vi "1_Counter_Time_Trace.vi"() -> ()   [LabVIEW 2015]
uses:
  C:/Users/MX-Microscope/Documents/LabVIEW Data/lvoop_campus_2018/Detector_Class/Swabian/time_tagger_vis/TTCSharp32.dll
  TTCSharp32.dll
panel:
  out "XY Graph 2":cluster{"Y":dbl[], "Y":dbl[]}[](graph)
  out "XY Graph":cluster{"Y":dbl[], "Y":dbl[]}[](graph)
  # "The built in test signal (~ 800 to 900 kHz) is applied first to channel 0 and 1 s later to channel 1."
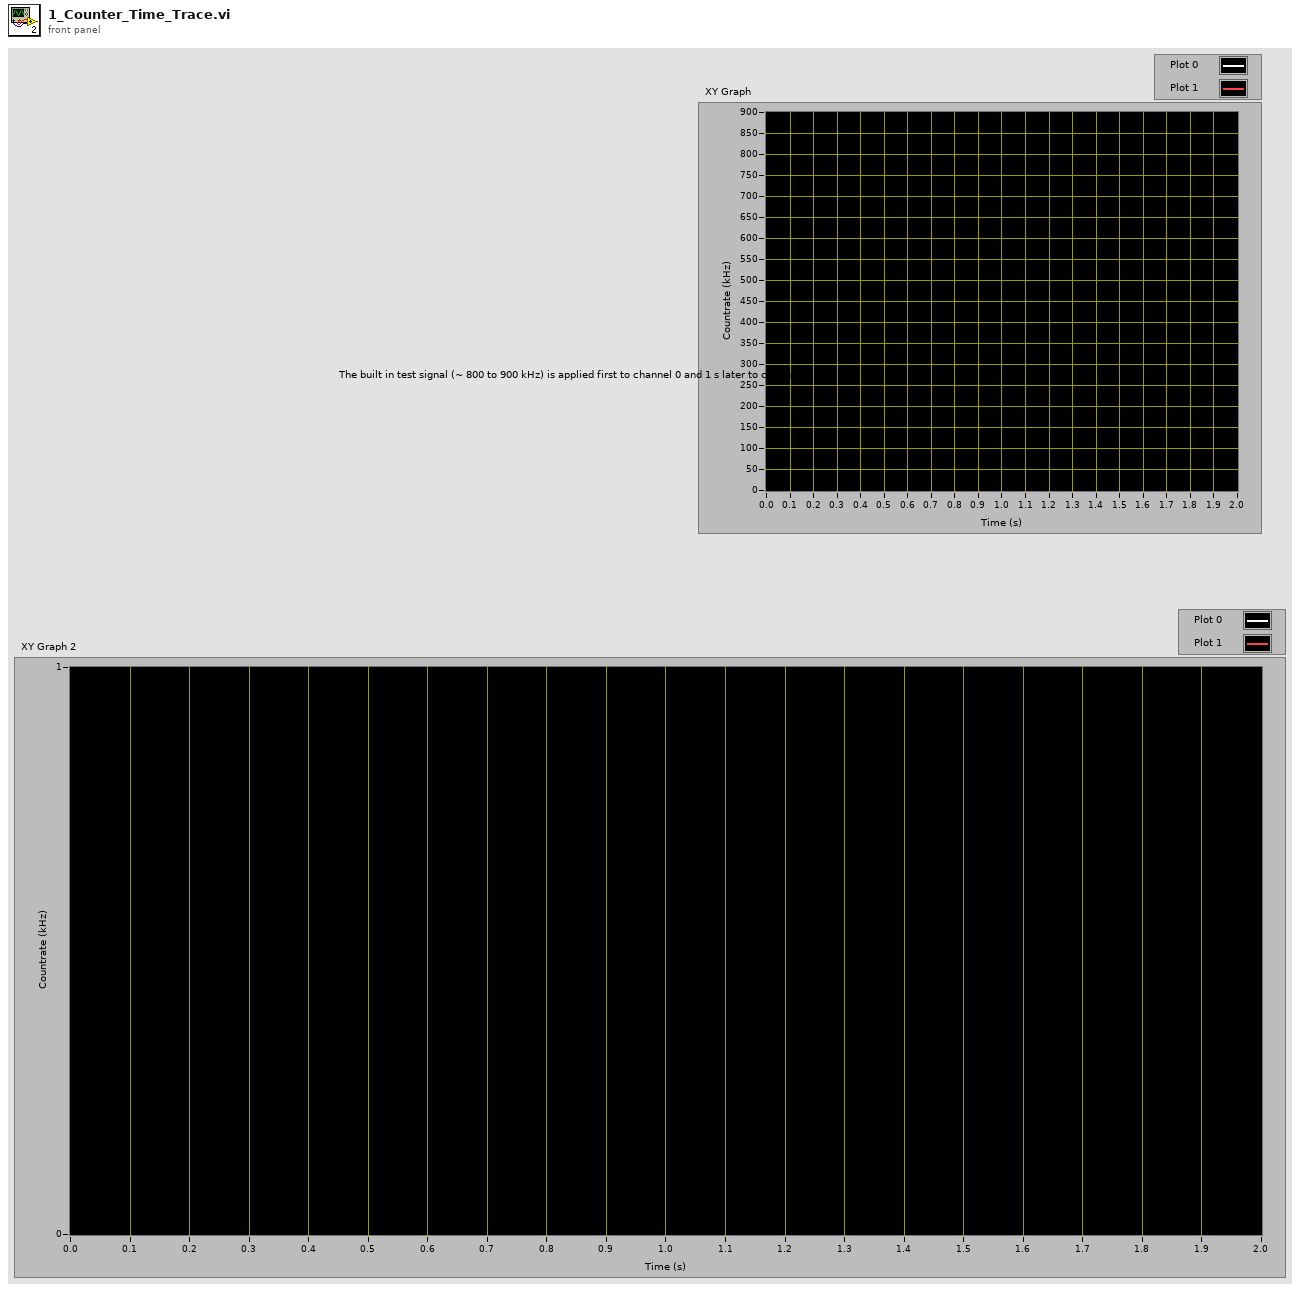
[diagram p1: front panel]
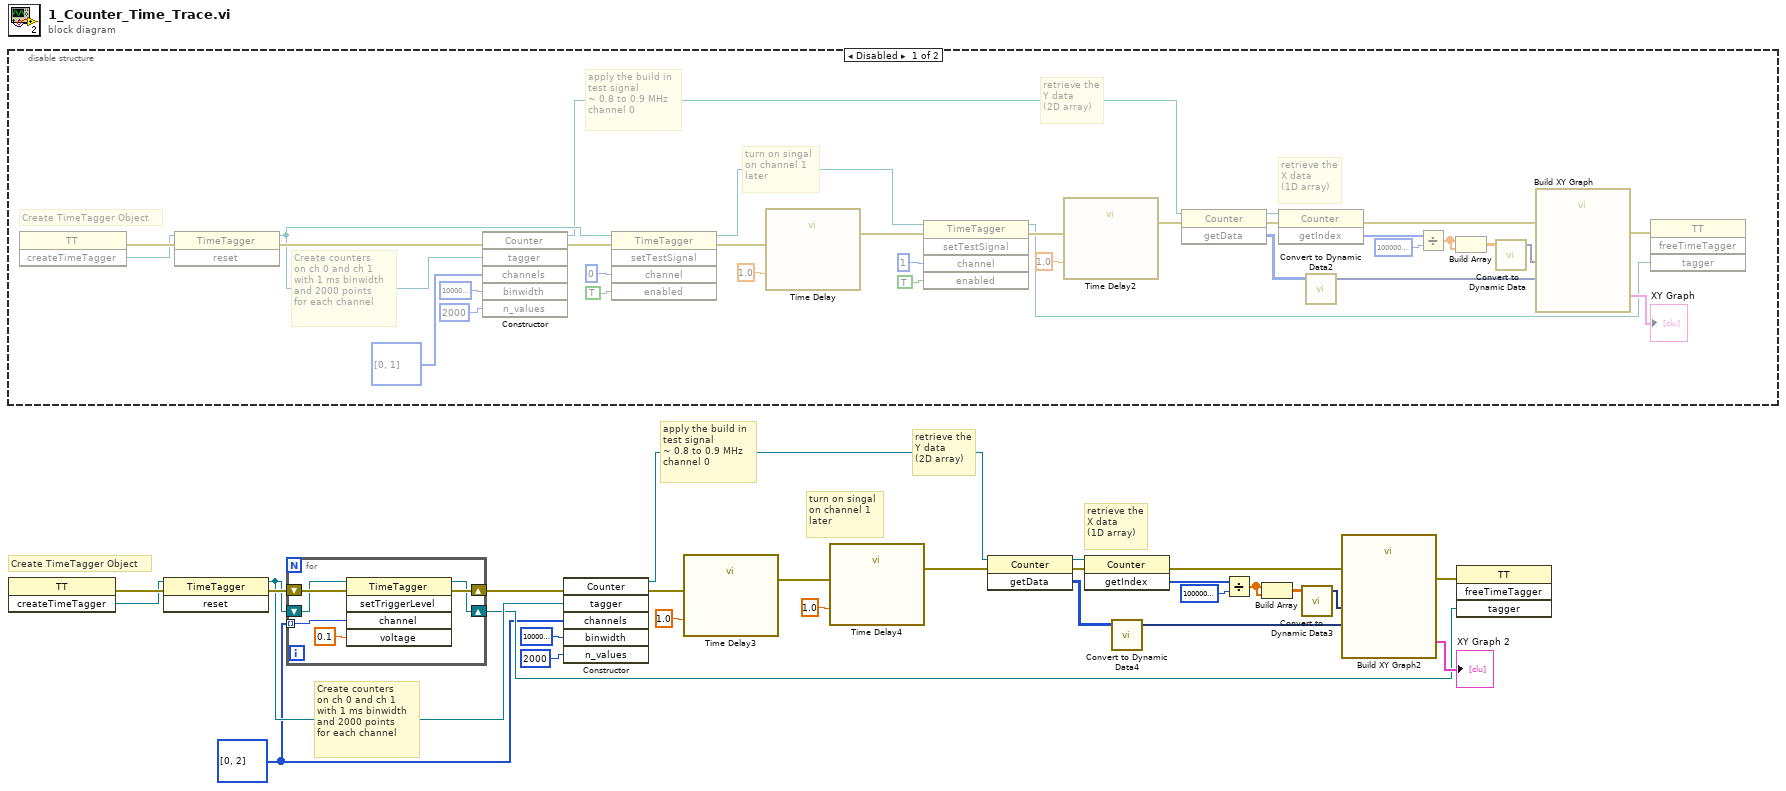
[diagram p0: block diagram]
diagram:
  w1 = u32[] [0, 2] ("channels")
  # "retrieve the\nX data\n(1D array)"
  # "retrieve the\nY data\n(2D array)"
  # "turn on singal\non channel 1\nlater"
  # "apply the build in\ntest signal\n~ 0.8 to 0.9 MHz\nchannel 0"
  # "Create counters\non ch 0 and ch 1\nwith 1 ms binwidth\nand 2000 points\nfor each channel"
  # "Create TimeTagger Object"
  n1 = disable-structure shown="Disabled" {
    frame Disabled {
      # "retrieve the\nX data\n(1D array)"
      # "retrieve the\nY data\n(2D array)"
      # "turn on singal\non channel 1\nlater"
      # "apply the build in\ntest signal\n~ 0.8 to 0.9 MHz\nchannel 0"
      # "Create counters\non ch 0 and ch 1\nwith 1 ms binwidth\nand 2000 points\nfor each channel"
      # "Create TimeTagger Object"
      n2 = invoke class="TT" method="createTimeTagger"() -> (error out=w56:errorcluster, "createTimeTagger"=w55:refnum<k24>)  [unwired: 3 in, 1 out]
      n3 = invoke class="TimeTagger" method="reset"(reference=w55, error in=w56) -> (reference out=w47:refnum<k24>, error out=w54:errorcluster)  [unwired: 1 in, 1 out]
      n4 = constructor class="Counter"(error in=w54, "tagger"=w47, "channels"=u32[] [0, 1], "binwidth"=i64 1000000000, "n_values"=2000) -> (reference out=w45:refnum<k24>, error out=w46:errorcluster)  [unwired: 2 in, 5 out]
      n5 = invoke class="TimeTagger" method="setTestSignal"(reference=w47, error in=w46, "channel"=u32 0, "enabled"=TRUE) -> (reference out=w48:refnum<k24>, error out=w50:errorcluster)  [unwired: 1 in, 3 out]
      n6 = call "Time Delay"("error in (no error)"=w50, "Delay Time (s)"=1.0) -> ("error out"=w49:errorcluster)  [unwired: 9 in]
      n7 = invoke class="TimeTagger" method="setTestSignal"(reference=w48, error in=w49, "channel"=u32 1, "enabled"=TRUE) -> (reference out=w28:refnum<k24>, error out=w43:errorcluster)  [unwired: 1 in, 3 out]
      n8 = call "Time Delay2"("error in (no error)"=w43, "Delay Time (s)"=1.0) -> ("error out"=w40:errorcluster)  [unwired: 9 in]
      n9 = invoke class="Counter" method="getData"(reference=w45, error in=w40) -> (reference out=w42:refnum<k24>, error out=w41:errorcluster, "getData"=w34:i32[][])  [unwired: 1 in]
      n10 = invoke class="Counter" method="getIndex"(reference=w42, error in=w41) -> (error out=w37:errorcluster, "getIndex"=w32:i64[])  [unwired: 1 in, 1 out]
      n11 = call "Convert to Dynamic Data2"("2D Array"=w34) -> ("Dynamic Data Type"=w33:dynamicdata)  [unwired: 3 in]
      n12 = Divide(x=w32, y=i64 1000000000000) -> (x/y=w31:dbl[])
      n13 = Build Array(w31, w31) -> (w36:dbl[][])
      n14 = call "Convert to Dynamic Data"("2D Array"=w36) -> ("Dynamic Data Type"=w35:dynamicdata)  [unwired: 3 in]
      n15 = call "Build XY Graph"("error in (no error)"=w37, "Y Input"=w33, "X Input"=w35) -> ("error out"=w29:errorcluster, "XY Graph"=→"XY Graph":cluster{"X":dbl[], "Y":dbl[]}[])  [unwired: 7 in]
      n16 = invoke class="TT" method="freeTimeTagger"(error in=w29, "tagger"=w28) -> ()  [unwired: 2 in, 4 out]
    }
    frame Enabled {
    }
  }
  n17 = invoke class="TT" method="createTimeTagger"() -> (error out=w27:errorcluster, "createTimeTagger"=w26:refnum<k24>)  [unwired: 3 in, 1 out]
  n18 = invoke class="TimeTagger" method="reset"(reference=w26, error in=w27) -> (reference out=w3:refnum<k24>, error out=w5:errorcluster)  [unwired: 1 in, 1 out]
  n19 = for {
    tunnel: w1 -> [w62] mode=indexing
    shift-right: [w65] -> w4
    shift-left: w5 -> [w66]
    shift-right: [w63] -> w2
    shift-left: w3 -> [w64]
    n20 = invoke class="TimeTagger" method="setTriggerLevel"(reference=w64, error in=w66, "channel"=w62, "voltage"=0.1) -> (reference out=w63:refnum<k24>, error out=w65:errorcluster)  [unwired: 1 in, 3 out]
  }
  n21 = constructor class="Counter"(error in=w4, "tagger"=w3, "channels"=w1, "binwidth"=i64 1000000000, "n_values"=2000) -> (reference out=w22:refnum<k24>, error out=w7:errorcluster)  [unwired: 2 in, 5 out]
  n22 = call "Time Delay3"("error in (no error)"=w7, "Delay Time (s)"=1.0) -> ("error out"=w6:errorcluster)  [unwired: 9 in]
  n23 = call "Time Delay4"("error in (no error)"=w6, "Delay Time (s)"=1.0) -> ("error out"=w18:errorcluster)  [unwired: 9 in]
  n24 = invoke class="Counter" method="getData"(reference=w22, error in=w18) -> (reference out=w20:refnum<k24>, error out=w19:errorcluster, "getData"=w13:i32[][])  [unwired: 1 in]
  n25 = invoke class="Counter" method="getIndex"(reference=w20, error in=w19) -> (error out=w16:errorcluster, "getIndex"=w11:i64[])  [unwired: 1 in, 1 out]
  n26 = call "Convert to Dynamic Data4"("2D Array"=w13) -> ("Dynamic Data Type"=w12:dynamicdata)  [unwired: 3 in]
  n27 = Divide(x=w11, y=i64 1000000000000) -> (x/y=w10:dbl[])
  n28 = Build Array(w10, w10) -> (w15:dbl[][])
  n29 = call "Convert to Dynamic Data3"("2D Array"=w15) -> ("Dynamic Data Type"=w14:dynamicdata)  [unwired: 3 in]
  n30 = call "Build XY Graph2"("error in (no error)"=w16, "Y Input"=w12, "X Input"=w14) -> ("error out"=w8:errorcluster, "XY Graph"=→"XY Graph 2":cluster{"X":dbl[], "Y":dbl[]}[])  [unwired: 7 in]
  n31 = invoke class="TT" method="freeTimeTagger"(error in=w8, "tagger"=w2) -> ()  [unwired: 2 in, 4 out]
